vi "Reset.vi"(8 "error in":errorcluster, 11 "fpga session in":refnum<k20>) -> (0 "error out":errorcluster, 3 "fpga session out":refnum<k20>)   [LabVIEW 2018, in "Lock-In Amplifier Example Host.lvlib"]
uses:
  Lock-In Amplifier Example Host.lvlib
  <instrlib>/_niInstr/Streaming/v1/Host/niInstr Streaming v1 Host.lvlib
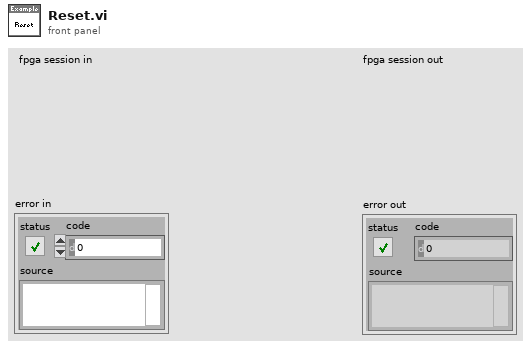
[diagram p1: front panel]
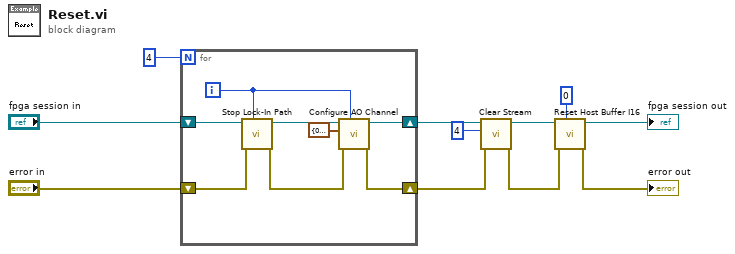
[diagram p0: block diagram]
diagram:
  n1 = for {
    N: 4 -> [_]
    shift-right: [w15] -> w5
    shift-left: "error in" -> [w18]
    shift-right: [w14] -> w8
    shift-left: "fpga session in" -> [w19]
    i -> [w13]
    n2 = call "Stop Lock-In Path.vi"("instance"=w13, "error in"=w18, "fpga session in"=w19) -> ("error out"=w16:errorcluster, "fpga session out"=w17:refnum<k20>)  [unwired: 7 in]
    n3 = call "Configure AO Channel.vi"("index"=w13, "error in"=w16, "config"=cluster{"carrier":dbl, "level":dbl} {"carrier"=0.0, "level"=0.0}, "fpga session in"=w17) -> ("error out"=w15:errorcluster, "fpga session out"=w14:refnum<k20>)  [unwired: 6 in]
  }
  n4 = call <instrlib>:"Clear Stream.vi"("error in (no error)"=w5, "stream index"=4, "refnum in"=w8) -> ("error out"=w4:errorcluster, "refnum out"=w6:refnum<k20>)  [unwired: 7 in]
  n5 = call "Reset Host Buffer I16.vi"("index"=0, "error in"=w4, "fpga session in"=w6) -> ("error out"=→"error out":errorcluster, "fpga session out"=→"fpga session out":refnum<k20>)  [unwired: 7 in]
